vi "Get Generic Slave Data.vi"(8 "error in (no error)":errorcluster caption="Fehler (Eingang, kein Fehler)", 11 "EtherCAT Slave In":T9 {"VS ref" format="%.0x"}) -> (0 "error out":errorcluster caption="Fehler (Ausgang)", 3 "EtherCAT Slave out":T1 {"I/O Output Data"."BD Refs"."Data Reference" format="%.0x"; "I/O Input Data"."BD Refs"."Data Reference" format="%.0x"; "I/O Output Vars"."VS ref" format="%.0x"; "I/O Imput Vars"."VS ref" format="%.0x"; "VS ref" format="%.0x"})   [LabVIEW 2016, in "Scan Engine Custom Device.lvlib"]
uses:
  Scan Engine Custom Device.lvlib
  <vilib>/NI Veristand/Custom Device API/Custom Device Item Ref.ctl
  Type Defs/Generic ECAT Slave Data Cluster.ctl
  Type Defs/Generic ECAT Slave IOV Cluster.ctl
  Type Defs/UDV Data Type.ctl
  Type Defs/Input Data.ctl
  <vilib>/NI Veristand/Custom Device API/Block Data Reference.ctl
  <vilib>/NI Veristand/Custom Device API/Data Reference.ctl
  Type Defs/Output Data.ctl
  <vilib>/NI Veristand/Custom Device API/Custom Device API.lvlib
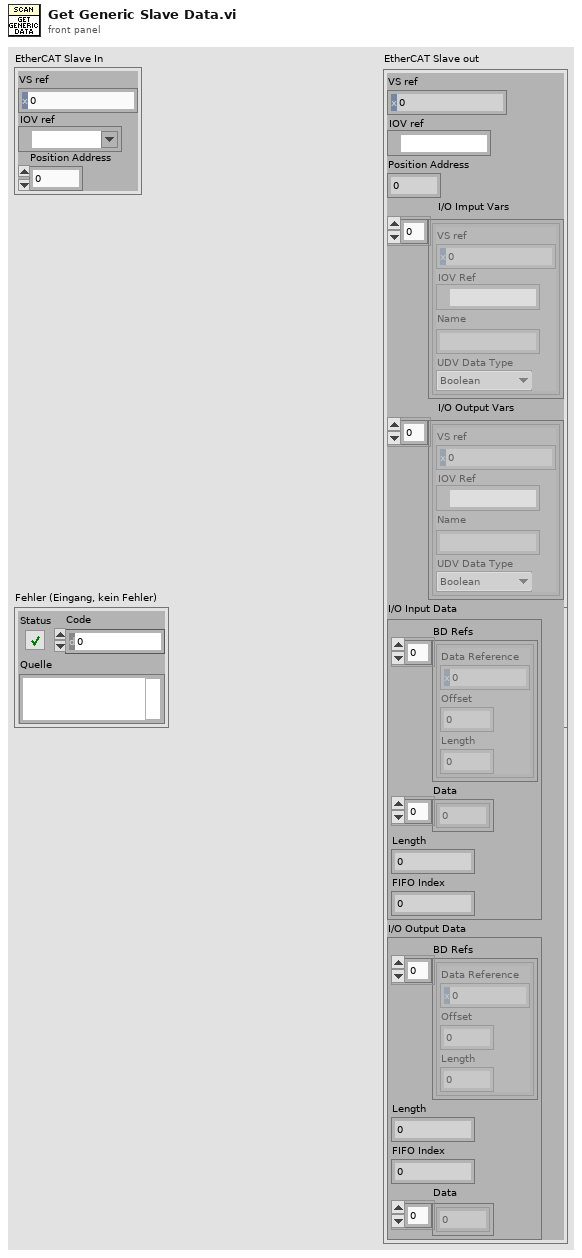
[diagram p1: front panel]
types:
  T1 = typedef "Scan Engine Custom Device.lvlib/Generic ECAT Slave Data Cluster.ctl" = cluster{"VS ref":T2, "IOV ref":refnum<k21>, "Position Address":u16, "I/O Imput Vars ":T3[], "I/O Output Vars":T3[], "I/O Input Data":T5, "I/O Output Data":T8}
  T2 = typedef "Custom Device API.lvlib/Custom Device Item Ref.ctl" = u64
  T3 = typedef "Scan Engine Custom Device.lvlib/Generic ECAT Slave IOV Cluster.ctl" = cluster{"VS ref":T2, "IOV Ref":refnum<k21>, "Name":string, "UDV Data Type":T4}
  T4 = typedef "Scan Engine Custom Device.lvlib/UDV Data Type.ctl" = enum16{"Boolean", "Fixed Point", "Int8", "Int16", "Int32", "Int64", "U32 Bit Field", "UInt8", "UInt16", "UInt32", "UInt64", "Other"}
  T5 = typedef "Scan Engine Custom Device.lvlib/Input Data.ctl" = cluster{"BD Refs":T6[], "Data":dbl[], "Length":i32, "FIFO Index":i32}
  T6 = typedef "Custom Device API.lvlib/Block Data Reference.ctl" = cluster{"Data Reference":T7, "Offset":u64, "Length":u64}
  T7 = typedef "Custom Device API.lvlib/Data Reference.ctl" = i32
  T8 = typedef "Scan Engine Custom Device.lvlib/Output Data.ctl" = cluster{"BD Refs":T6[], "Length":i32, "FIFO Index":i32, "Data":dbl[]}
  T9 = cluster{"VS ref":T2, "IOV ref":refnum<k21>, "Position Address":u16}
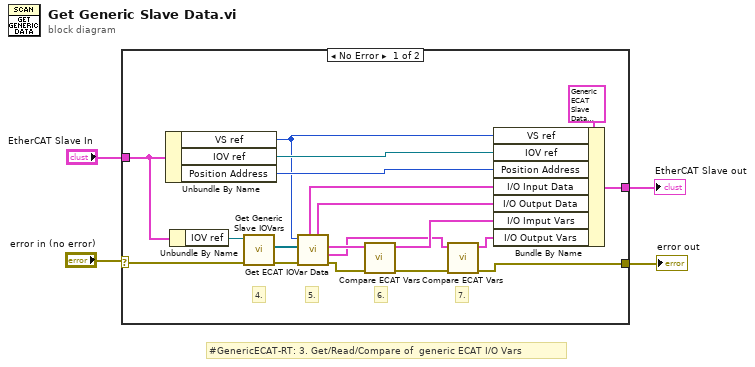
[diagram p0: block diagram]
diagram:
  # "#GenericECAT-RT: 3. Get/Read/Compare of  generic ECAT I/O Vars"
  n1 = case shown="No Error" "error in (no error)" {
    selector: "error in (no error)" -> [w23 w24]
    tunnel: "EtherCAT Slave In" -> [w21 _]
    tunnel: [w11 w24] -> w2
    tunnel: [w19 _] -> w1
    frame No Error {
      # "7."
      # "6."
      # "5."
      # "4."
      n2 = Unbundle By Name(w21) -> ("VS ref"=w14:T2, "IOV ref"=w15:refnum<k21>, "Position Address"=w20:u16)
      n3 = Unbundle By Name(w21) -> ("IOV ref"=w17:refnum<k21>)
      n4 = call "Get Generic Slave IOVars.vi"("error in (no error)"=w23, "ECAT Slave in"=w17) -> ("error IO"=w18:errorcluster, "ECAT Variablenobjekt"=w16:refnum<k21>[])  [unwired: 7 in, 1 out]
      n5 = call "Get ECAT IOVar Data.vi"("Fehler (Eingang, kein Fehler)"=w18, "ECAT Variablenobjekt"=w16, "VS ref"=w14) -> ("Fehler (Ausgang)"=w13:errorcluster, "I/O Output Vars"=w5:T3[], "I/O Imput Vars"=w8:T3[], "I/O Output Data"=w9:T8, "I/O Input Data"=w10:T5)  [unwired: 3 in, 1 out]
      n6 = call "Compare ECAT Vars.vi"("Fehler (Eingang, kein Fehler)"=w13, "I/O Output Vars (Eingang)"=w8) -> ("Fehler (Ausgang)"=w12:errorcluster, "I/O Output Vars (Ausgang)"=w7:T3[])  [unwired: 8 in]
      n7 = call "Compare ECAT Vars.vi"("Fehler (Eingang, kein Fehler)"=w12, "I/O Output Vars (Eingang)"=w5) -> ("Fehler (Ausgang)"=w11:errorcluster, "I/O Output Vars (Ausgang)"=w6:T3[])  [unwired: 8 in]
      n8 = Bundle By Name(cluster=T1 {"VS ref"=0, "IOV ref"="", "Position Address"=0, "I/O Imput Vars "=[], "I/O Output Vars"=[], "I/O Input Data"={"BD Refs"=[], "Data"=[], "Length"=0, "FIFO Index"=0}, "I/O Output Data"={"BD Refs"=[], "Length"=0, "FIFO Index"=0, "Data"=[]}} ("EtherCAT Slave"), "VS ref"=w14, "IOV ref"=w15, "Position Address"=w20, "I/O Input Data"=w10, "I/O Output Data"=w9, "I/O Imput Vars"=w7, "I/O Output Vars"=w6) -> (w19:T1)
    }
    frame Error {
    }
  }
  "error out" <- w2
  "EtherCAT Slave out" <- w1
